vi "B7_65_WriteAndCheck.vi"(0 "DriverConnect in":T1={"InterfaceType"=enum."VISA", "OpenedSession"="", "InterfaceSettings"={"Interface"=enum."RS232", "EOS 4 read"=enum."LF (\\n)", "EOS 4 write"=enum."LF (\\n)", "TMO, ms"=10000, "Sett"=variant(cluster{"Baud Rate":u32, "Data Bits":u16, "Parity":u16, "Stop Bits":u16, "Flow Control":u16, "Eho":bool} {"Baud Rate"=75, "Data Bits"=0, "Parity"=0, "Stop Bits"=0, "Flow Control"=0, "Eho"=FALSE})}}, 1 "Str2Write":string, 2 "Str2Check":string, 3 "Command Time (s)":T6=3, 11 "error in":T9, 12 "TMO, ms":T6=500, 13 "Driver Name":T7="B1_28", 14 "Error Code":T6=5490) -> (4 "DriverConnect out":T1={"InterfaceType"=enum."VISA", "OpenedSession"="", "InterfaceSettings"={"Interface"=enum."RS232", "EOS 4 read"=enum."LF (\\n)", "EOS 4 write"=enum."LF (\\n)", "TMO, ms"=10000, "Sett"=variant(cluster{"Baud Rate":u32, "Data Bits":u16, "Parity":u16, "Stop Bits":u16, "Flow Control":u16, "Eho":bool} {"Baud Rate"=75, "Data Bits"=0, "Parity"=0, "Stop Bits"=0, "Flow Control"=0, "Eho"=FALSE})}}, 15 "error out":T9)   [LabVIEW 2018]
uses:
  MOKO_LabViewLibrary/MokoLowLevel/MokoLowLovelControl/MLLC_Error.ctl
  MOKO_LabViewLibrary/MokoLowLevel/MokoLowLovelControl/MLLC_Response.ctl
  MOKO_LabViewLibrary/MokoLowLevel/MokoLowLovelControl/MLLC_DriverName.ctl
  MOKO_LabViewLibrary/MokoLowLevel/MokoLowLovelControl/MLLC_ErrorCode.ctl
  MOKO_LabViewLibrary/MokoLowLevel/MokoLowLovelControl/MLLC_ConnectCluster.ctl
  MOKO_LabViewLibrary/MokoLowLevel/MokoLowLovelControl/MLLC_InterfaceType.ctl
  MOKO_LabViewLibrary/MokoLowLevel/MokoLowLovelControl/MLLC_OpenedSession.ctl
  MOKO_LabViewLibrary/MokoLowLevel/MokoLowLovelControl/MLLC_InterfaceSettings.ctl
  MOKO_LabViewLibrary/MokoLowLevel/MokoLowLovelControl/MLLC_InterfaceKind.ctl
panel:
  out "Response RS232":T8
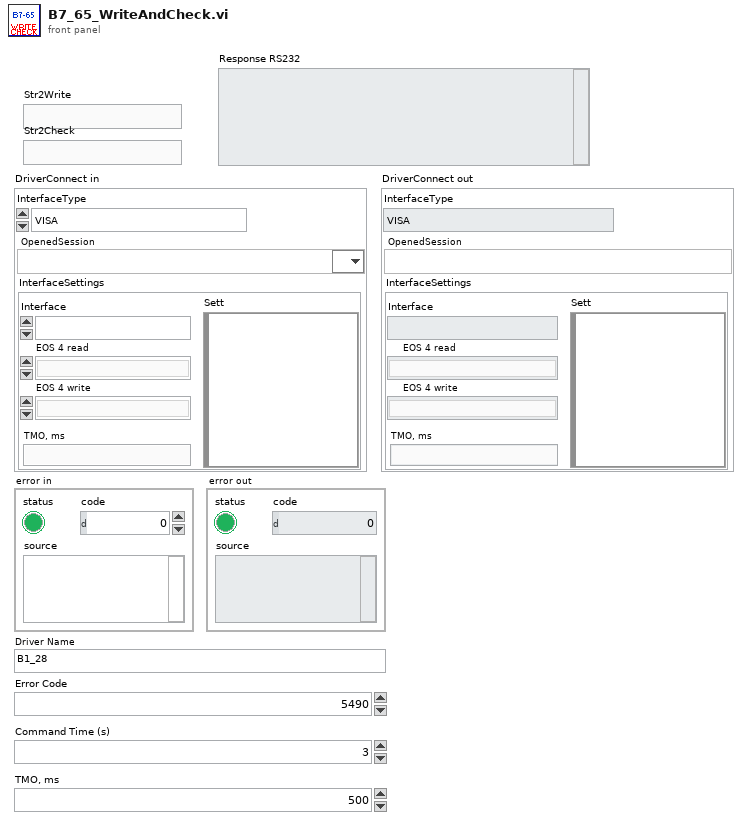
[diagram p1: front panel]
types:
  T1 = typedef "MLLC_ConnectCluster.ctl" = cluster{"InterfaceType":T2, "OpenedSession":T3, "InterfaceSettings":T4}
  T2 = typedef "MLLC_InterfaceType.ctl" = enum16{"VISA", "Prologix USB-GPIB"}
  T3 = typedef "MLLC_OpenedSession.ctl" = refnum<visa-resource-name>
  T4 = typedef "MLLC_InterfaceSettings.ctl" = cluster{"Interface":T5, "EOS 4 read":enum16{"Default (=EOS 4 write)", "CR (\\r)", "LF (\\n)", "None"}, "EOS 4 write":enum16{"CR+LF (\\r\\n)", "CR (\\r)", "LF (\\n)", "None"}, "TMO, ms":i32, "Sett":variant}
  T5 = typedef "MLLC_InterfaceKind.ctl" = enum16{"RS232", "GPIB", "USB", "Ethernet", "another"}
  T6 = typedef "MLLC_ErrorCode.ctl" = u32
  T7 = typedef "MLLC_DriverName.ctl" = string
  T8 = typedef "MLLC_Response.ctl" = string
  T9 = typedef "MLLC_Error.ctl" = errorcluster
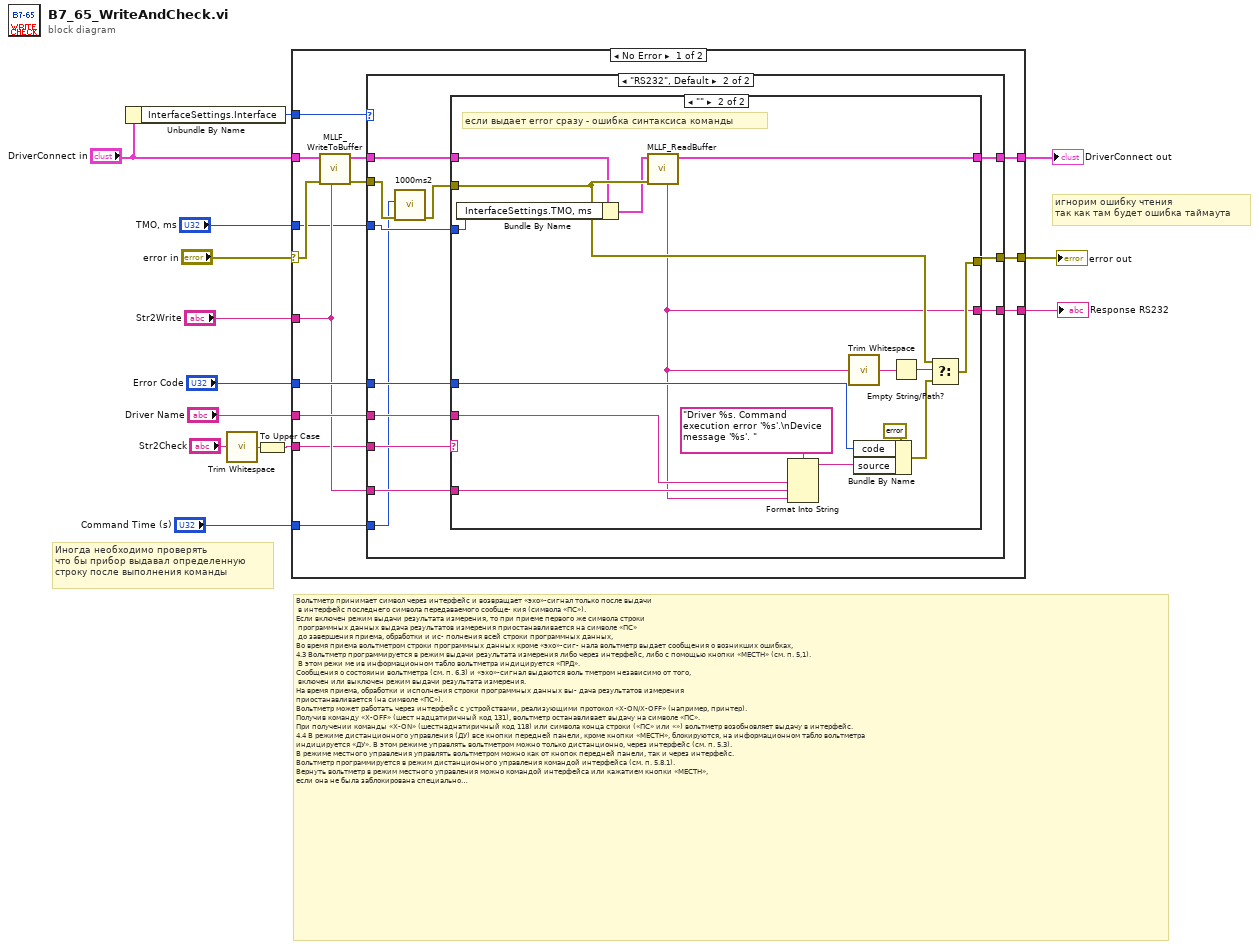
[diagram p0: block diagram]
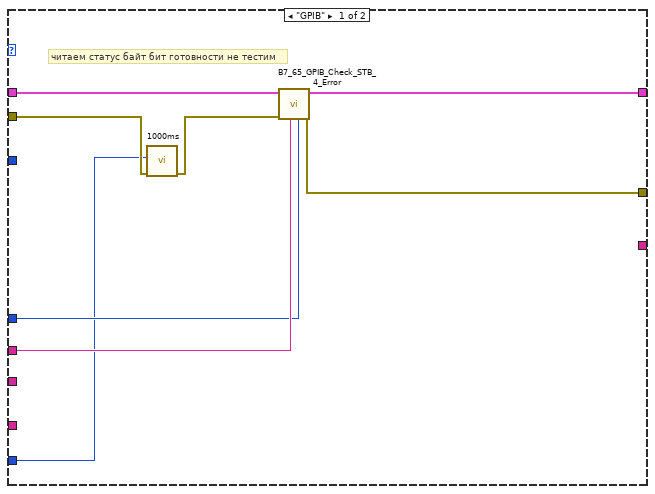
[diagram p2: hidden frame]
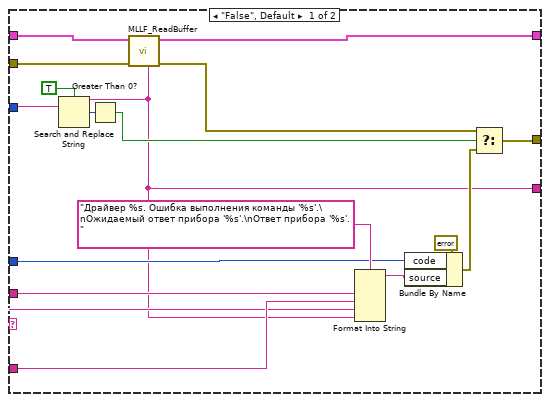
[diagram p3: hidden frame]
diagram:
  # "Вольтметр принимает символ через интерфейс и возвращает «эхо»-сигнал только после выдачи\n в интерфейс последнего символа передаваемого сообще- кия (символа «ПС»).\nЕсли включен режим выдачи результата измерения, то при приеме первого же символа строки\n программных данных выдача результатов измерения приостанавливается на символе «ПС»\n до завершения приема, обработки и ис- полнения всей строки программных данных,\nВо время приема вольтметром строки программных данных кроме «эхо»-сиг- нала вольтметр выдает сообщения о возникших ошибках,\n4.3 Вольтметр программируется в режим выдачи результата измерения либо через интерфейс, либо с помощью кнопки «МЕСТН» (см. п. 5,1).\n В этом режи ме ив информационном табло вольтметра индицируется «ПРД».\nСообщения о состояини вольтметра (см. п. 6.3) и «эхо»-сигнал выдаются воль тметром независимо от того,\n включен или выключен режим выдачи результата измерения.\nНа время приема, обработки и исполнения строки программных данных вы- дача результатов измерения \nприостанавливается (на символе «ПС»).\nВольтметр может работать через интерфейс с устройствами, реализующими протокол «Х-ON/X-OFF» (например, принтер). \nПолучив команду «X-OFF» (шест надцатиричный код 131), вольтметр останавливает выдачу на символе «ПС». \nПри получении команды «X-ON» (шестнаднатиричный код 118) или символа конца строки («ПС» или «») вольтметр возобновляет выдачу в интерфейс.\n4.4 В режиме дистанционного управления (ДУ) все кнопки передней панели, кроме кнопки «МЕСТН», блокируются, на информационном табло вольтметра \nиндицируется «ДУ». В этом режиме управлять вольтметром можно только дистанционно, через интерфейс (см. п. 5.3).\nВ режиме местного управления управлять вольтметром можно как от кнопок передней панели, так и через интерфейс.\nВольтметр программируется в режим дистанционного управления командой интерфейса (см. п. 5.8.1). \nВернуть вольтметр в режим местного управления можно командой интерфейса или кажатием кнопки «МЕСТН», \nесли она не была заблокирована специальной командой интерфейса (см. п. 5.8.2).\nФункции кнопки «МЕСТН» в режиме местного управления описаны в п. 5. 1."
  # "Иногда необходимо проверять \nчто бы прибор выдавал определенную\nстроку после выполнения команды"
  # "игнорим ошибку чтения\nтак как там будет ошибка таймаута"
  n1 = Unbundle By Name("DriverConnect in") -> ("InterfaceSettings.Interface"=w4:T5)
  n2 = call <vilib>:"Trim Whitespace.vi"("string"="Str2Check") -> ("trimmed string"=w8:string)  [unwired: 1 in]
  n3 = To Upper Case(1:w8) -> (0:w6:string)
  n4 = case shown="No Error" "error in" {
    selector: "error in" -> [w28 w83]
    tunnel: [w21 w83] -> w14
    tunnel: [w26 w82] -> w1
    tunnel: "Str2Write" -> [w22 _]
    tunnel: "Error Code" -> [w24 _]
    tunnel: "Driver Name" -> [w23 _]
    tunnel: w6 -> [w20 _]
    tunnel: [w19 _] -> w9
    tunnel: "TMO, ms" -> [w18 _]
    tunnel: w4 -> [w17 _]
    tunnel: "Command Time (s)" -> [w16 _]
    tunnel: "DriverConnect in" -> [w15 w82]
    frame No Error {
      n5 = call "MLLF_WriteToBuffer.vi"("String"=w22, "error in"=w28, "DriverConnect in"=w15) -> ("error out"=w25:T9, "DriverConnect out"=w27:T1)  [unwired: 5 in]
      n6 = case shown="\"RS232\", Default" w17 {
        tunnel: w27 -> [w36 w48]
        tunnel: [w32 w47] -> w26
        tunnel: w25 -> [w30 w39]
        tunnel: w24 -> [w34 w46]
        tunnel: w23 -> [w35 w45]
        tunnel: w22 -> [_ w44]
        tunnel: [w33 w43] -> w21
        tunnel: w20 -> [_ w42]
        tunnel: [_ w41] -> w19
        tunnel: w18 -> [_ w40]
        tunnel: w16 -> [w29 w37]
        frame "GPIB" {
          # "читаем статус байт бит готовности не тестим"
          n7 = call "1000ms"("error in (no error)"=w30, "Delay Time (s)"=w29) -> ("error out"=w31:errorcluster)  [unwired: 9 in]
          n8 = call "B7_65_GPIB_Check_STB_4_Error.vi"("Error Code"=w34, "Driver Name"=w35, "error in"=w31, "DriverConnect in"=w36) -> ("error out"=w33:T9, "DriverConnect out"=w32:T1)  [unwired: 6 in]
        }
        frame "RS232", Default {
          n9 = call "1000ms2"("error in (no error)"=w39, "Delay Time (s)"=w37) -> ("error out"=w38:errorcluster)  [unwired: 9 in]
          n10 = case shown="\"\"" w42 {
            selector: w42 -> [w50 _]
            tunnel: w48 -> [w64 w67]
            tunnel: [w54 w81] -> w47
            tunnel: w38 -> [w65 w78]
            tunnel: w46 -> [w53 w73]
            tunnel: w45 -> [w52 w72]
            tunnel: w44 -> [w51 w71]
            tunnel: [w55 w70] -> w43
            tunnel: [w49 w69] -> w41
            tunnel: w40 -> [_ w68]
            frame "False", Default {
              n11 = call "MLLF_ReadBuffer.vi"("Error In"=w65, "DriverConnect in"=w64) -> ("Error Out"=w60:errorcluster, "DriverConnect out"=w54:T1, "String"=w49:string)  [unwired: 6 in]
              n12 = Search and Replace String(case sensitive?=TRUE ("ignore case? (F)"), input string=w49, search string=w50) -> (number of replacements=w62:i32)  [unwired: 5 in, 3 out]
              n13 = Greater Than 0?(x=w62) -> (x > 0?=w61:bool)
              n14 = Format Into String(format string="Драйвер %s. Ошибка выполнения команды '%s'.\nОжидаемый ответ прибора '%s'.\nОтвет прибора '%s'. ", w52, w51, w50, w49) -> (resulting string=w59:string)  [unwired: 2 in, 1 out]
              n15 = Bundle By Name(cluster=errorcluster {"status"=TRUE, "code"=5100, "source"="B1-28. Timeout."} ("error in"), "code"=w53, "source"=w59) -> (w56:errorcluster)
              n16 = Select(t=w60, s=w61, f=w56) -> (s? t:f=w55:errorcluster)
            }
            frame "" {
              # "если выдает error сразу - ошибка синтаксиса команды"
              n17 = Bundle By Name(cluster=w67, "InterfaceSettings.TMO, ms"=w68) -> (w66:T1)
              n18 = call "MLLF_ReadBuffer.vi"("Error In"=w78, "DriverConnect in"=w66) -> ("DriverConnect out"=w81:T1, "String"=w69:string)  [unwired: 6 in, 1 out]
              n19 = Format Into String(format string="Driver %s. Command execution error '%s'.\nDevice message '%s'. ", w72, w71, w69) -> (resulting string=w75:string)  [unwired: 2 in, 1 out]
              n20 = call <vilib>:"Trim Whitespace.vi"("string"=w69) -> ("trimmed string"=w80:string)  [unwired: 1 in]
              n21 = Bundle By Name(cluster=errorcluster {"status"=TRUE, "code"=5100, "source"="B1-28. Timeout."} ("error in"), "code"=w73, "source"=w75) -> (w74:errorcluster)
              n22 = Empty String/Path?(string/path=w80) -> (empty?=w79:bool)
              n23 = Select(t=w78, s=w79, f=w74) -> (s? t:f=w70:errorcluster)
            }
          }
        }
      }
    }
    frame Error {
    }
  }
  "error out" <- w14
  "Response RS232" <- w9
  "DriverConnect out" <- w1
